vi "GetRegisterArray.vi"(8 "error in (no error)":errorcluster, 11 "JSON Text":string) -> (0 "error out":errorcluster, 3 "Register Array":string[](array[string]) caption="<JSON>Elements")   [LabVIEW 2017]
uses:
  <vilib>/JDP Science/JSONtext/JSONtext.lvlib
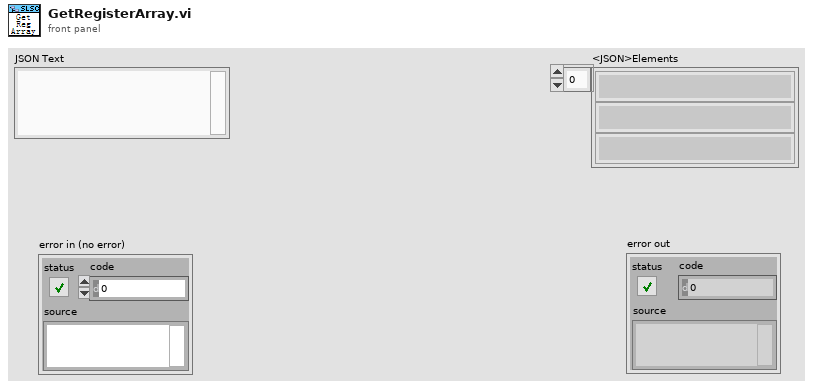
[diagram p1: front panel]
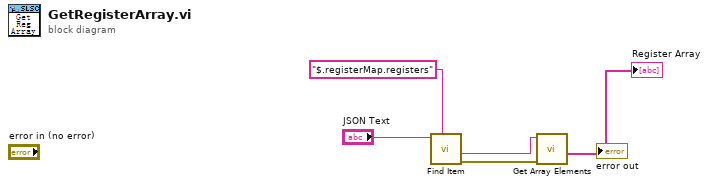
[diagram p0: block diagram]
diagram:
  n1 = call <vilib>:"Find Item.vi"("$Path or Item Name"="$.registerMap.registers", "JSON"="JSON Text") -> ("error out"=w2:errorcluster, "<JSON>"=w3:string)  [unwired: 6 in, 2 out]
  n2 = call <vilib>:"Get Array Elements.vi"("error in (no error)"=w2, "JSON"=w3) -> ("<JSON>"=→"Register Array":string[])  [unwired: 7 in, 2 out]
